vi "Do.vi"(8 "error in (no error)":errorcluster, 10 "Actor in":refnum<class "Actor.lvclass">, 11 "Wait Msg":refnum<class "Wait Msg.lvclass">) -> (0 "error out":errorcluster, 2 "Actor out":refnum<class "Actor.lvclass">)   [LabVIEW 2020, in "Sequencer.lvlib" / "Wait Msg.lvclass"]
doc: "Call the Stop Msg Do method to stop the Sequencer actor."
uses:
  Wait Msg.lvclass
  PPL/HDH.Actor Framework.Core.Actor.lvlibp/1abvi3w/vi.lib/ActorFramework/Actor/Actor.lvclass
  Sequencer/Sequencer.lvclass
  C:/Current projects/WS/PPL/HDH.Actor Framework.Core.Actor.lvlibp/1abvi3w/vi.lib/ActorFramework/Actor/Actor.lvclass
  Wait Msg.lvclass/Wait Msg.ctl
  Sequencer/Sequencer.lvclass/Sequencer.ctl
  Sequencer Core/Sequencer Core.lvclass/Sequencer Core.ctl
  PPL/HDH.Data.Generic.lvlibp/Synchronization/Notifier/Wait Single.vi
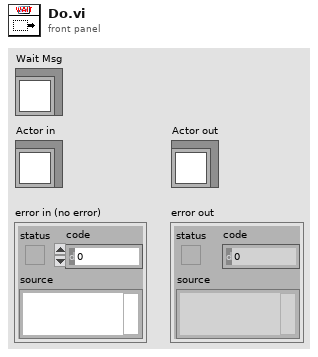
[diagram p1: front panel]
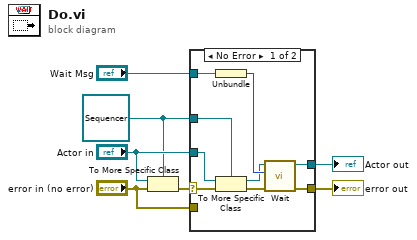
[diagram p0: block diagram]
diagram:
  w1 = refnum<class "Sequencer.lvclass"> refnum ("Sequencer.lvlib:Sequencer.lvclass")
  n1 = To More Specific Class(target class=w1, reference="Actor in", error in="error in (no error)") -> (error out=w7:errorcluster)  [unwired: 1 out]
  n2 = case shown="No Error" w7 {
    selector: w7 -> [w14 _]
    tunnel: [w10 w17] -> w6
    tunnel: "Actor in" -> [w12 w17]
    tunnel: [w8 w18] -> w4
    tunnel: "error in (no error)" -> [_ w18]
    tunnel: "Wait Msg" -> [w16 _]
    tunnel: w1 -> [w13 _]
    frame No Error {
      n3 = Unbundle(w16) -> (w15:i32)
      n4 = To More Specific Class(target class=w13, reference=w12, error in=w14) -> (specific class reference=w11:refnum<class "Sequencer.lvclass">, error out=w9:errorcluster)
      n5 = call "Wait.vi"("error in (no error)"=w9, "Timeout in ms (0)"=w15, "Sequencer in"=w11) -> ("error out"=w8:errorcluster, "Sequencer out"=w10:refnum<class "Sequencer.lvclass">)  [unwired: 6 in, 1 out]
    }
    frame Error {
    }
  }
  "error out" <- w4
  "Actor out" <- w6
